vi "FFT Output BRAM Ping Pong Control Logic.vi"(8 "Input Valid":bool, 10 "Read Count":u16, 11 "Write Count":u16) -> (0 "Read Valid":bool, 1 "BRAM Bank0 Write?":bool, 2 "Read Address 2":u16, 3 "Read Address1":u16)   [LabVIEW 2011]
uses:
  <instrlib>/FlexRIO/Libraries/Helper VIs/NI FlexRIO Helper VIs.lvlib
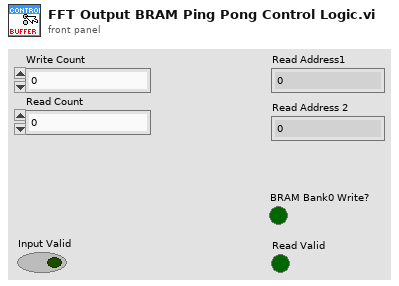
[diagram p1: front panel]
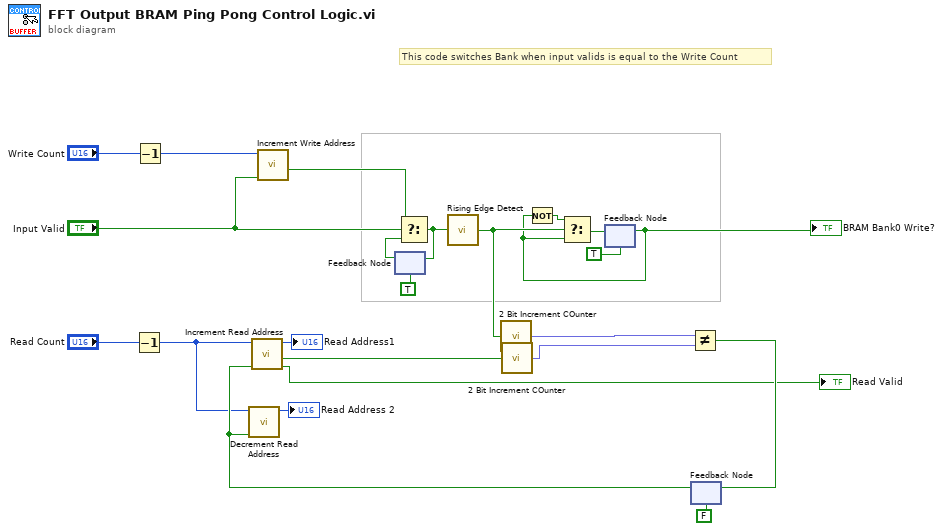
[diagram p0: block diagram]
diagram:
  # "This code switches Bank when input valids is equal to the Write Count"
  n1 = Decrement(x="Read Count") -> (x-1=w2:u16)
  n2 = Decrement(x="Write Count") -> (x-1=w6:u16)
  n3 = call <userlib>:"Increment Write Address.vi"("INC?"="Input Valid", "rollover"=w6) -> ("roll over"=w17:bool)  [unwired: 7 in, 2 out]
  n4 = feedback #1(TRUE ("roll over")) -> (w16:bool)
  n5 = Select(t=w17, s="Input Valid", f=w16) -> (s? t:f=w15:bool)
  n6 = feedback-in #1(w15) -> ()
  n7 = call <instrlib>:"Rising Edge Detect.vi"("signal"=w15) -> ("edge detected"=w18:bool)  [unwired: 14 in]
  n8 = call <userlib>:"2 Bit Increment COunter.vi"("Increment"=w18) -> ("Counter Value"=w22:fxp<+,3,3>)  [unwired: 14 in]
  n9 = feedback #2(TRUE) -> (w9:bool)
  "BRAM Bank0 Write?" <- w9
  n10 = Not(x=w9) -> (.not. x?=w19:bool)
  n11 = Select(t=w19, s=w18, f=w9) -> (s? t:f=w13:bool)
  n12 = feedback-in #2(w13) -> ()
  n13 = feedback #3(FALSE) -> (w3:bool)
  n14 = call <userlib>:"Decrement Read Address.vi"("DEC?"=w3, "Load Value"=w2) -> ("count"=→"Read Address 2":u16)  [unwired: 8 in, 1 out]
  n15 = call <userlib>:"Increment Read Address.vi"("INC?"=w3, "rollover"=w2) -> ("Output Valid"=→"Read Valid":bool, "roll over"=w23:bool, "count"=→"Read Address1":u16)  [unwired: 7 in]
  n16 = call <userlib>:"2 Bit Increment COunter.vi"("Increment"=w23) -> ("Counter Value"=w20:fxp<+,3,3>)  [unwired: 14 in]
  n17 = Not Equal?(x=w22, y=w20) -> (x != y?=w11:bool)
  n18 = feedback-in #3(w11) -> ()
